vi "RequestLEDAction.vi"(8 "Height Setpoint":dbl, 11 "Action":T1) -> ()   [LabVIEW 2018]
uses:
  Actions.ctl
  LEDSetpoint.vi
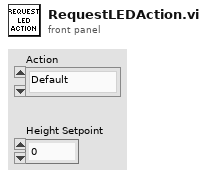
[diagram p1: front panel]
types:
  T1 = typedef "Actions.ctl" = enum16{"Default", "Hatch Triggered", "Lost Vision", "Auto Aiming", "Party Mode", "Has Hatch", "Brownout", "Height Setpoint"}
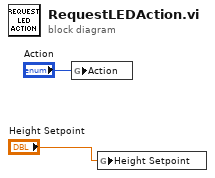
[diagram p0: block diagram]
diagram:
  n1 = global write "LEDSetpoint.vi" "Action"("Action") -> ()
  n2 = global write "LEDSetpoint.vi" "Height Setpoint"("Height Setpoint") -> ()
